vi "Check for New Floor Tile.vi"(2 "Bounds":T1, 3 "Current Location":cdb) -> (0 "Add floor tile ?":bool, 1 "New Floor Tile":cdb)   [LabVIEW 2020, in "AoC 2022.lvlib"]
uses:
  AoC 2022.lvlib
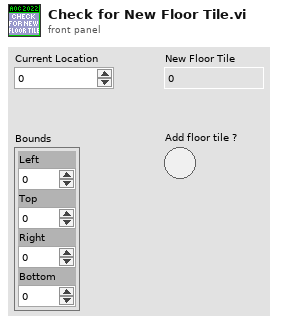
[diagram p1: front panel]
types:
  T1 = cluster{"Left":i16, "Top":i16, "Right":i16, "Bottom":i16}
  T2 = cluster{"Left":dbl, "Top":dbl, "Right":dbl, "Bottom":dbl}
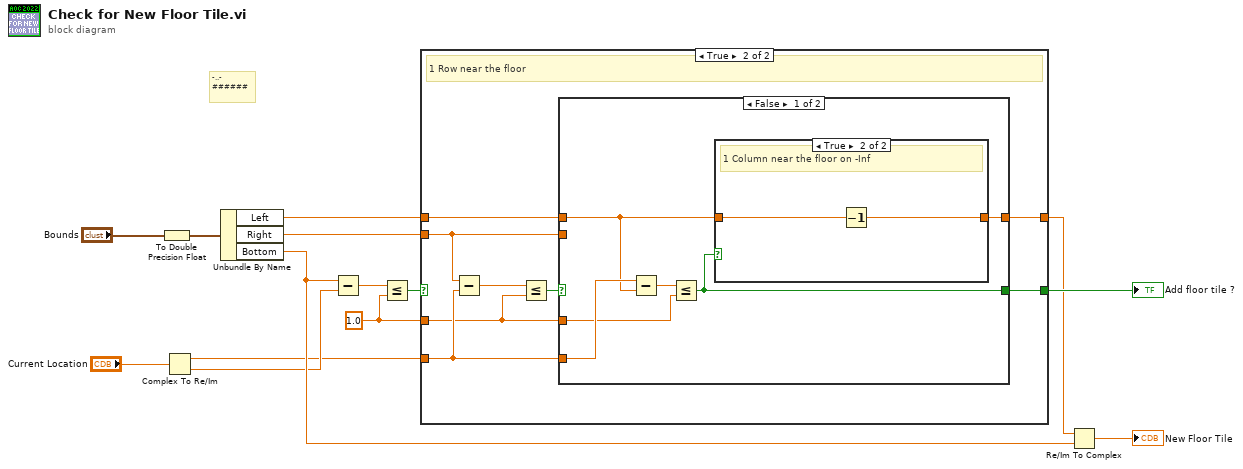
[diagram p0: block diagram]
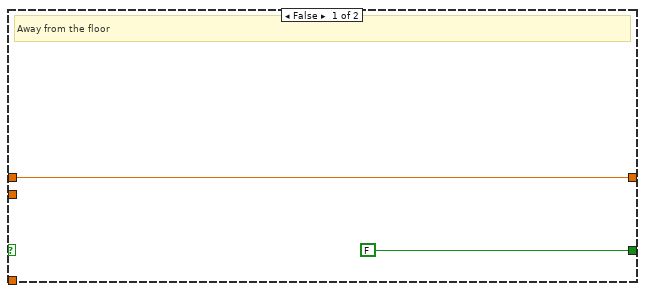
[diagram p2: hidden frame]
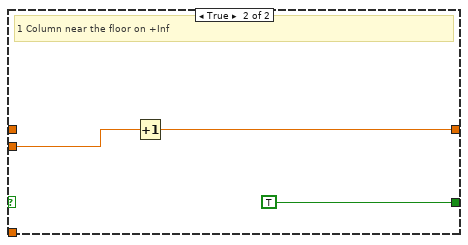
[diagram p4: hidden frame]
diagram:
  w7 = 1.0
  # "-..-\n######"
  n1 = To Double Precision Float(number="Bounds") -> (double precision float=w13:T2)
  n2 = Complex To Re/Im(x + iy="Current Location") -> (x=w1:dbl, y=w2:dbl)
  n3 = Unbundle By Name(w13) -> ("Left"=w8:dbl, "Right"=w9:dbl, "Bottom"=w5:dbl)
  n4 = Subtract(x=w5, y=w2) -> (x-y=w11:dbl)
  n5 = Less Or Equal?(x=w11, y=w7) -> (x <= y?=w10:bool)
  n6 = case shown="True" w10 {
    tunnel: w9 -> [_ w17]
    tunnel: w1 -> [_ w21]
    tunnel: w8 -> [w15 w22]
    tunnel: w7 -> [_ w20]
    tunnel: [FALSE w19] -> w6
    tunnel: [w15 w18] -> w3
    frame False {
      # "Away from the floor"
    }
    frame True {
      # "1 Row near the floor"
      n7 = Subtract(x=w17, y=w21) -> (x-y=w24:dbl)
      n8 = Less Or Equal?(x=w24, y=w20) -> (x <= y?=w23:bool)
      n9 = case shown="False" w23 {
        tunnel: w22 -> [w25 _]
        tunnel: w21 -> [w30 _]
        tunnel: w20 -> [w28 _]
        tunnel: [w27 TRUE] -> w19
        tunnel: [w26 w35] -> w18
        tunnel: w17 -> [_ w34]
        frame False {
          n10 = Subtract(x=w30, y=w25) -> (x-y=w29:dbl)
          n11 = Less Or Equal?(x=w29, y=w28) -> (x <= y?=w27:bool)
          n12 = case shown="True" w27 {
            tunnel: w25 -> [w31 w33]
            tunnel: [w31 w32] -> w26
            frame False {
              # "Away from the boundary"
            }
            frame True {
              # "1 Column near the floor on -Inf"
              n13 = Decrement(x=w33) -> (x-1=w32:dbl)
            }
          }
        }
        frame True {
          # "1 Column near the floor on +Inf"
          n14 = Increment(x=w34) -> (x+1=w35:dbl)
        }
      }
    }
  }
  "Add floor tile ?" <- w6
  n15 = Re/Im To Complex(1:w5, 2:w3) -> (0:→"New Floor Tile":cdb)
